vi "getTrace_.vi"(5 "ptr":u32, 6 "Buffer":string, 7 "Trace attribute IN":T1) -> (1 "Array":dbl[](array[numeric]), 3 "Trace attribute OUT":T1)   [LabVIEW 2017, in "HEKAdat.lvclass"]
uses:
  HEKAdat.lvclass
panel:
  out "Waveform":dbl[](graph)
  out "Datascaler":dbl format="%#_6e"
  out "Unit":string
  out "Xinterval":dbl format="%#_6e"
  out "label":string
  out "nDatapoints":u32
  out "offset":u32
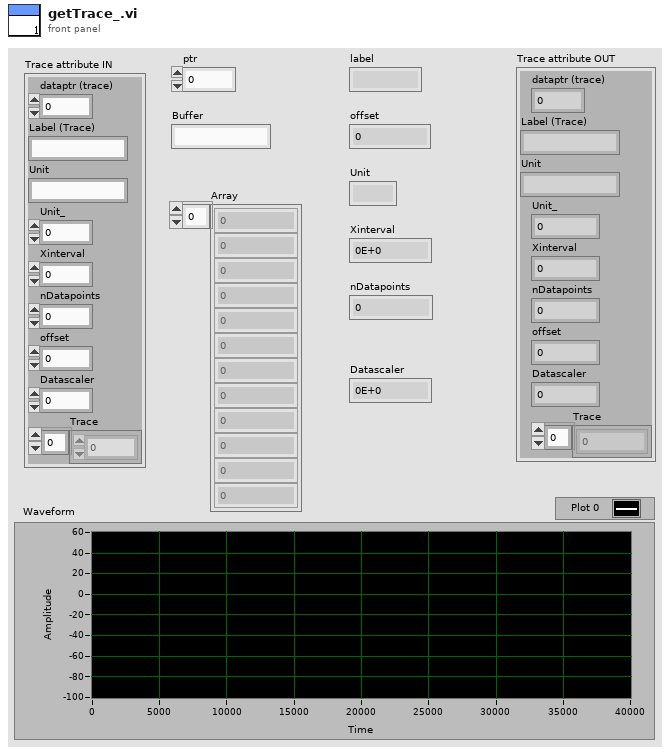
[diagram p1: front panel]
types:
  T1 = cluster{"dataptr (trace)":u32, "Label (Trace)":string, "Unit":string, "Unit_":dbl, "Xinterval":dbl, "nDatapoints":u32, "offset":u32, "Datascaler":dbl, "Trace":dbl[]}
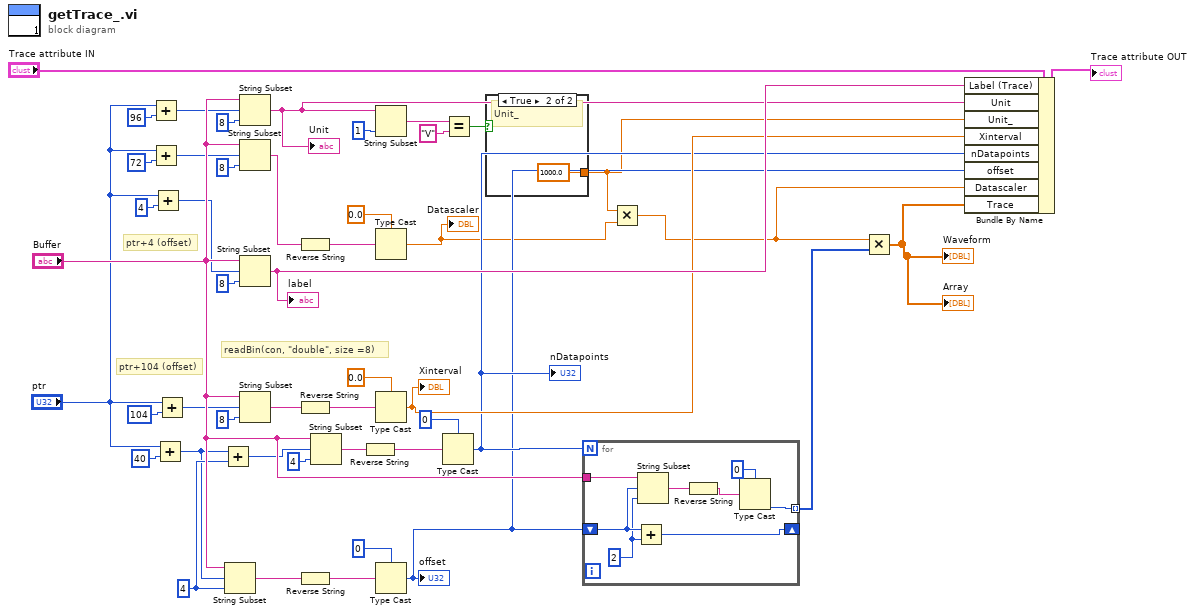
[diagram p0: block diagram]
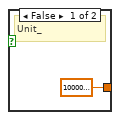
[diagram p2: hidden frame]
diagram:
  w21 = u32 4 ("length (rest)")
  # "readBin(con, \"double\", size =8)"
  # "ptr+104 (offset)"
  # "ptr+4 (offset)"
  n1 = Add(x="ptr", y=u32 96 ("length (rest)")) -> (x+y=w37:u32)
  n2 = Add(x="ptr", y=u32 72 ("length (rest)")) -> (x+y=w40:u32)
  n3 = Add(x="ptr", y=u32 4 ("length (rest)")) -> (x+y=w22:u32)
  n4 = Add(x="ptr", y=u32 40 ("length (rest)")) -> (x+y=w20:u32)
  n5 = Add(x="ptr", y=u32 104 ("length (rest)")) -> (x+y=w27:u32)
  n6 = Add(x=w20, y=w21) -> (x+y=w32:u32)
  n7 = String Subset(string="Buffer", offset (0)=w20, length (rest)=w21) -> (substring=w13:string)
  n8 = String Subset(string="Buffer", offset (0)=w37, length (rest)=u32 8 ("length (rest)")) -> (substring=w9:string)
  "Unit" <- w9
  n9 = String Subset(string="Buffer", offset (0)=w40, length (rest)=u32 8 ("length (rest)")) -> (substring=w44:string)
  n10 = String Subset(string="Buffer", offset (0)=w22, length (rest)=u32 8 ("length (rest)")) -> (substring=w10:string)
  "label" <- w10
  n11 = String Subset(string="Buffer", offset (0)=w27, length (rest)=u32 8 ("length (rest)")) -> (substring=w30:string)
  n12 = Reverse String(1:w44) -> (0:w43:string)
  n13 = Reverse String(1:w30) -> (0:w28:string)
  n14 = Reverse String(1:w13) -> (0:w12:string)
  n15 = String Subset(string="Buffer", offset (0)=w32, length (rest)=4 ("length (rest)")) -> (substring=w18:string)
  n16 = Reverse String(1:w18) -> (0:w19:string)
  n17 = String Subset(string=w9, length (rest)=1 ("length (rest)")) -> (substring=w35:string)  [unwired: 1 in]
  n18 = Type Cast(type=0.0, x=w43) -> (*(type *) &x=w2:dbl)
  "Datascaler" <- w2
  n19 = Type Cast(type=0.0, x=w28) -> (*(type *) &x=w8:dbl)
  "Xinterval" <- w8
  n20 = Type Cast(type=u32 0, x=w12) -> (*(type *) &x=w6:u32)
  "offset" <- w6
  n21 = Type Cast(type=u32 0, x=w19) -> (*(type *) &x=w7:u32)
  "nDatapoints" <- w7
  n22 = Equal?(x=w35, y="V") -> (x = y?=w34:bool)
  n23 = case shown="True" w34 {
    tunnel: [1000000000.0 ("xinterval 2") 1000.0 ("xinterval 2")] -> w4
    frame False {
      # "Unit_"
    }
    frame True {
      # "Unit_"
    }
  }
  n24 = for {
    N: w7 -> [_]
    tunnel: "Buffer" -> [w56]
    tunnel: [w52] -> w47 mode=indexing
    shift-right: [w53] -> _
    shift-left: w6 -> [w55]
    w54 = u32 2 ("length (rest)")
    n25 = Add(x=w55, y=w54) -> (x+y=w53:u32)
    n26 = String Subset(string=w56, offset (0)=w55, length (rest)=w54) -> (substring=w51:string)
    n27 = Reverse String(1:w51) -> (0:w50:string)
    n28 = Type Cast(type=i16 0, x=w50) -> (*(type *) &x=w52:i16)
  }
  n29 = Multiply(x=w4, y=w2) -> (x*y=w1:dbl)
  n30 = Multiply(x=w1, y=w47) -> (x*y=w3:dbl[])
  "Waveform" <- w3
  "Array" <- w3
  n31 = Bundle By Name(cluster="Trace attribute IN", "Label (Trace)"=w10, "Unit"=w9, "Unit_"=w4, "Xinterval"=w8, "nDatapoints"=w7, "offset"=w6, "Datascaler"=w1, "Trace"=w3) -> (→"Trace attribute OUT":T1)
